vi "GetVariableFromFile.vi"(9 "variableFileName":string, 10 "Ftp":refnum<k24>, 11 "error in":errorcluster) -> (2 "Variables":T1(array[cluster]), 3 "error out":errorcluster)   [LabVIEW 2016, in "UnderAutomation.Fanuc.lvlib"]
uses:
  UnderAutomation.Fanuc.lvlib
  C:/Users/fg/Documents/Fanuc.vi/LabVIEW_2024/UnderAutomation.Fanuc/lib/UnderAutomation.Fanuc.dll
  LabVIEW_2024/UnderAutomation.Fanuc/lib/UnderAutomation.Fanuc.dll
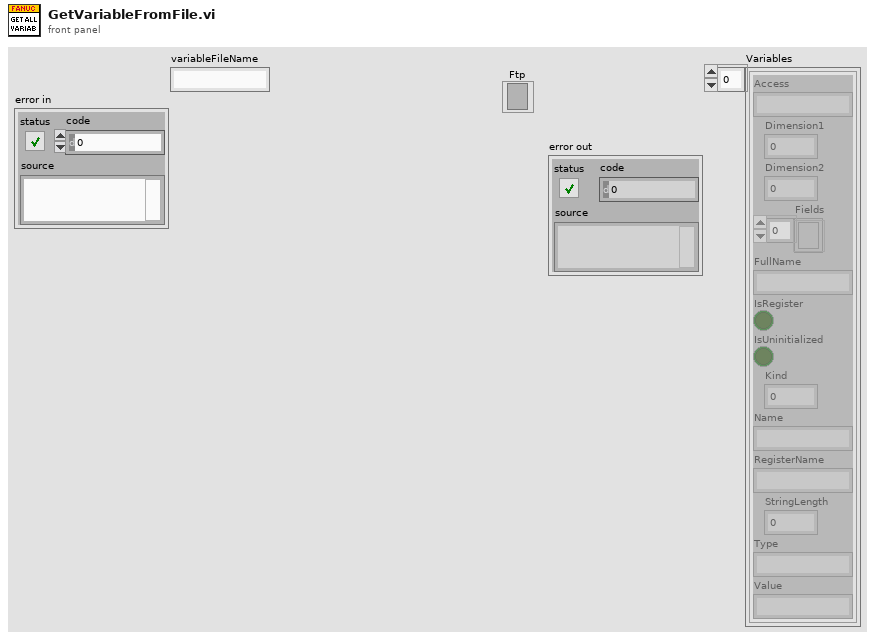
[diagram p1: front panel]
types:
  T1 = cluster{"Access":string, "Dimension1":i32, "Dimension2":i32, "Fields":refnum<k24>[], "FullName":string, "IsRegister":bool, "IsUninitialized":bool, "Kind":i32, "Name":string, "RegisterName":string, "StringLength":i32, "Type":string, "Value":string}[]
  T2 = cluster{"Access":string, "Dimension1":i32, "Dimension2":i32, "Fields":refnum<k24>[], "FullName":string, "IsRegister":bool, "IsUninitialized":bool, "Kind":i32, "Name":string, "RegisterName":string, "StringLength":i32, "Type":string, "Value":string}
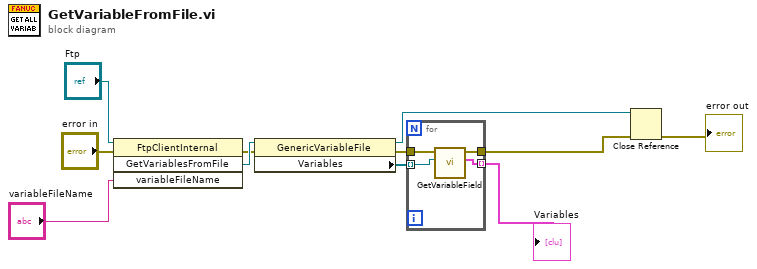
[diagram p0: block diagram]
diagram:
  n1 = invoke class="FtpClientInternal" method="GetVariablesFromFile"(reference="Ftp", error in="error in", "variableFileName"="variableFileName") -> (error out=w4:errorcluster, "GetVariablesFromFile"=w8:refnum<k24>)  [unwired: 1 in, 2 out]
  n2 = property class="GenericVariableFile"(reference=w8, error in=w4) -> (reference out=w1:refnum<k24>, error out=w5:errorcluster, "Variables"=w7:refnum<k24>[])
  n3 = for {
    tunnel: w7 -> [w15] mode=indexing
    tunnel: [w14] -> w6 mode=indexing
    tunnel: w5 -> [w13]
    tunnel: [w12] -> w3
    n4 = call "GetVariableField.vi"("Field"=w15, "error in (no error)"=w13) -> ("Field cluster"=w14:T2, "error out"=w12:errorcluster)  [unwired: 8 in]
  }
  "Variables" <- w6
  n5 = Close Reference(reference=w1, error in (no error)=w3) -> (error out=→"error out":errorcluster)
